vi "Write Analyze Fluence Obj.vi"(8 "error in (no error)":errorcluster, 10 "Analyze.lvlib:Analyze Fluence.lvclass":refnum<class "Analyze Fluence.lvclass">, 11 "Analyze Fluence and Energy in":refnum<class "Analyze Fluence and Energy.lvclass">) -> (0 "error out":errorcluster, 3 "Analyze Fluence and Energy out":refnum<class "Analyze Fluence and Energy.lvclass">)   [LabVIEW 2014, in "Analyze.lvlib" / "Analyze Fluence and Energy.lvclass"]
uses:
  Analyze Fluence and Energy.lvclass
  Analyze Fluence/Analyze Fluence.lvclass
  Analyze Fluence and Energy.lvclass/Analyze Fluence and Energy.ctl
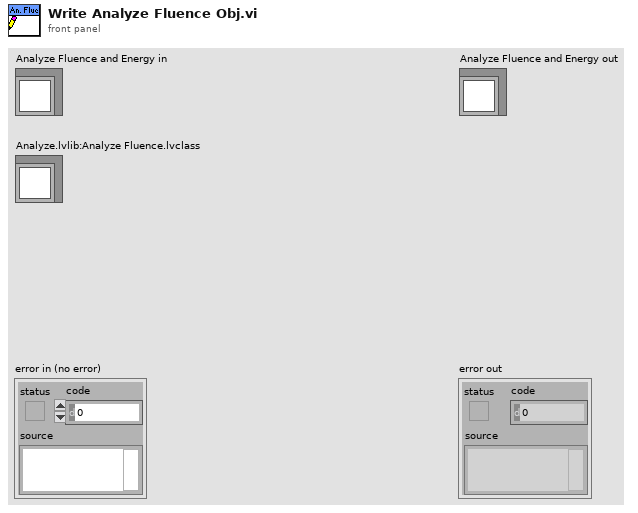
[diagram p1: front panel]
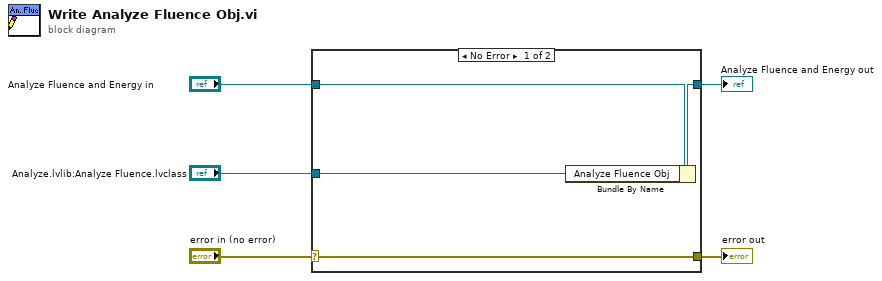
[diagram p0: block diagram]
diagram:
  n1 = case shown="No Error" "error in (no error)" {
    selector: "error in (no error)" -> [w9 w10]
    tunnel: [w9 w10] -> w4
    tunnel: [w7 w11] -> w2
    tunnel: "Analyze Fluence and Energy in" -> [w8 w11]
    tunnel: "Analyze.lvlib:Analyze Fluence.lvclass" -> [w6 _]
    frame No Error {
      n2 = Bundle By Name(cluster=w8, "Analyze Fluence Obj"=w6) -> (w7:refnum<class "Analyze Fluence and Energy.lvclass">)
    }
    frame Error {
    }
  }
  "error out" <- w4
  "Analyze Fluence and Energy out" <- w2
